vi "XY Graph Get Last Plot ID.vi"(8 "error in (no error)":errorcluster, 11 "XYGraph in":refnum<vi>) -> (0 "error out":errorcluster, 1 "Last Plot ID":i32, 3 "XYGraph out":refnum<vi>)   [LabVIEW 2021, in "XY Graph Add-Ons.lvlib"]
uses:
  XY Graph Add-Ons.lvlib
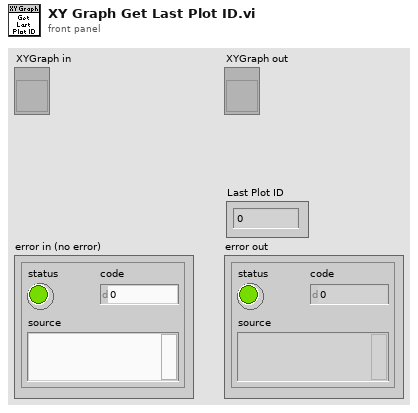
[diagram p1: front panel]
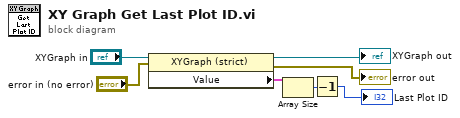
[diagram p0: block diagram]
diagram:
  n1 = property class="XYGraph (strict)"(reference="XYGraph in", error in="error in (no error)") -> (reference out=→"XYGraph out":refnum<vi>, error out=→"error out":errorcluster, "Value"=w3:cluster{dbl[], dbl[]}[])
  n2 = Array Size(array=w3) -> (size(s)=w2:i32)
  n3 = Decrement(x=w2) -> (x-1=→"Last Plot ID":i32)
